vi "CfgManager.Text Test Launcher.vi"() -> ()   [LabVIEW 2013]
uses:
  Manager/ConfigManager.lvclass
  Manager/ConfigManager.lvclass/ConfigManager.ctl
  Serializer/Serializer.lvclass
  Encoding/Encoding.lvclass
  Encryption/Encryption.lvclass
  Manager.Text/ConfigManager.Text.lvclass
  Manager/Write.vi
  Manager/Read Serializer.vi
  Manager/Read Encoding.vi
  Manager/Read Encryption.vi
  Manager/Decompose KVPs.vi
  Manager/Read.vi
  <vilib>/LabVIEW Open Source/Data Manipulation/KVP Parser.vi
  <vilib>/Utility/VariantDataType/GetTypeInfo.vi
panel:
  out "Keys":string[](array[string])
  out "post-modified value":variant
  out "error out":errorcluster
  out "pre-modified value":variant
  in  "filepath":path
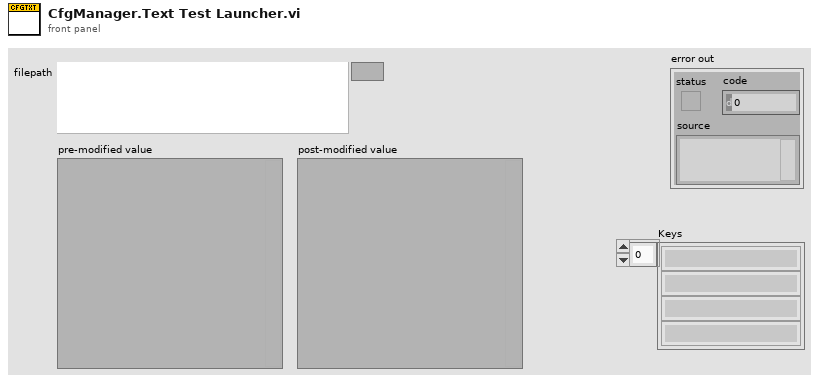
[diagram p1: front panel]
types:
  T1 = cluster{"String":string, "Numeric":dbl, "Boolean":bool}
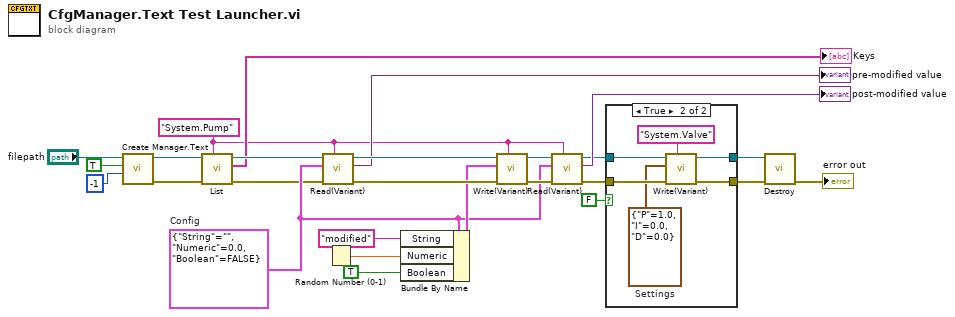
[diagram p0: block diagram]
diagram:
  w6 = "System.Pump" ("Qualified Name")
  w18 = T1 {"String"="", "Numeric"=0.0, "Boolean"=FALSE}  # Config
  n1 = call "Create Manager.Text.vi"("write delay (ms)"=-1, "save on destroy (T)"=TRUE, "filepath"="filepath") -> ("error out"=w13:errorcluster, "ConfigManager.Text out"=w14:refnum<class "ConfigManager.Text.lvclass">)  [unwired: 7 in]
  n2 = call "List.vi"("Qualified Name"=w6, "error in (no error)"=w13, "ConfigManager in"=w14) -> ("error out"=w12:errorcluster, "Keys"=→"Keys":string[], "ConfigManager out"=w11:refnum<class "ConfigManager.Text.lvclass">)  [unwired: 6 in]
  n3 = call "Read(Variant).vi"("Qualified Name"=w6, "error in (no error)"=w12, "Type"=w18, "ConfigManager in"=w11) -> ("error out"=w23:errorcluster, "value"=→"pre-modified value":variant, "ConfigManager out"=w24:refnum<class "ConfigManager.Text.lvclass">)  [unwired: 3 in, 2 out]
  n4 = Random Number (0-1)() -> (number: 0 to 1=w22:dbl)
  n5 = Bundle By Name(cluster=w18, "String"="modified", "Numeric"=w22, "Boolean"=TRUE) -> (w21:T1)
  n6 = call "Write(Variant).vi"("Qualified Name"=w6, "error in (no error)"=w23, "value"=w21, "ConfigManager in"=w24) -> ("error out"=w19:errorcluster, "ConfigManager out"=w20:refnum<class "ConfigManager.Text.lvclass">)  [unwired: 5 in, 1 out]
  n7 = call "Read(Variant).vi"("Qualified Name"=w6, "error in (no error)"=w19, "Type"=w18, "ConfigManager in"=w20) -> ("error out"=w3:errorcluster, "value"=→"post-modified value":variant, "ConfigManager out"=w5:refnum<class "ConfigManager.Text.lvclass">)  [unwired: 3 in, 2 out]
  n8 = case shown="True" FALSE {
    tunnel: w5 -> [w28 w34]
    tunnel: [w28 w33] -> w4
    tunnel: w3 -> [w27 w32]
    tunnel: [w27 w31] -> w2
    frame False {
    }
    frame True {
      w29 = cluster{"P":dbl, "I":dbl, "D":dbl} {"P"=1.0, "I"=0.0, "D"=0.0}  # Settings
      n9 = call "Write(Variant).vi"("Qualified Name"="System.Valve", "error in (no error)"=w32, "value"=w29, "ConfigManager in"=w34) -> ("error out"=w31:errorcluster, "ConfigManager out"=w33:refnum<class "ConfigManager.Text.lvclass">)  [unwired: 5 in, 1 out]
    }
  }
  n10 = call-dynamic "Destroy.vi"("error in (no error)"=w2, "ConfigManager.Text in"=w4) -> ("error out"=→"error out":errorcluster)  [unwired: 8 in, 1 out]
